vi "subset.vi"() -> ()   [LabVIEW 2019]
panel:
  out "substring":string
  in  "string":string="Butterfly"
  # "This program will make a new substring"
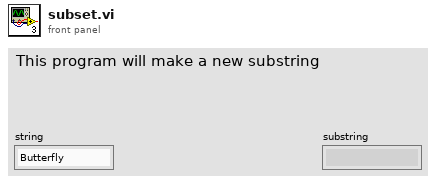
[diagram p1: front panel]
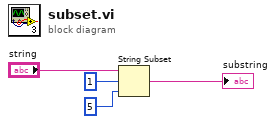
[diagram p0: block diagram]
diagram:
  n1 = String Subset(string="string", offset (0)=1, length (rest)=5 ("offset (0)")) -> (substring=→"substring":string)
